vi "Calculate New Velocity.vi"(6 "Acceleration":sgl, 8 "Sin Heading":sgl, 9 "Cos Heading":sgl, 10 "Current Velocity y":sgl, 11 "Current Velocity x":sgl) -> (2 "New Velocity y":sgl, 3 "New Velocity x":sgl)   [LabVIEW 2015, in "Math.lvlib"]
uses:
  Math.lvlib
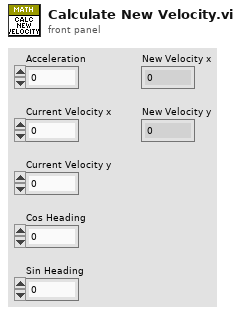
[diagram p1: front panel]
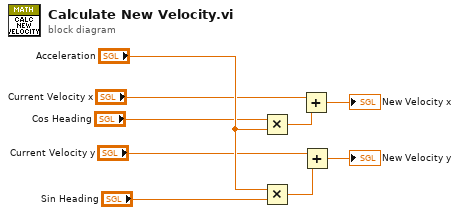
[diagram p0: block diagram]
diagram:
  n1 = Multiply(x="Cos Heading", y="Acceleration") -> (x*y=w3:sgl)
  n2 = Multiply(x="Acceleration", y="Sin Heading") -> (x*y=w5:sgl)
  n3 = Add(x="Current Velocity x", y=w3) -> (x+y=→"New Velocity x":sgl)
  n4 = Add(x="Current Velocity y", y=w5) -> (x+y=→"New Velocity y":sgl)
